vi "Read Pre AIV Values.vi"(8 "error in":errorcluster, 11 "DAC HeatFlow AIV in":refnum<class "DAC HeatFlow AIV.lvclass">) -> (0 "error out":errorcluster, 3 "DAC HeatFlow AIV out":refnum<class "DAC HeatFlow AIV.lvclass">)   [LabVIEW 2019, in "DAC.lvlib" / "DAC HeatFlow AIV.lvclass"]
uses:
  DAC HeatFlow AIV.lvclass
  <vilib>/DAQmx/read.llb/DAQmx Read (Analog DBL 1Chan 1Samp).vi
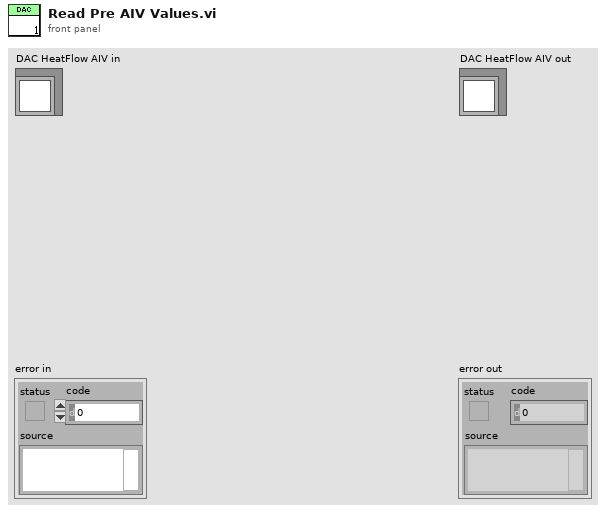
[diagram p1: front panel]
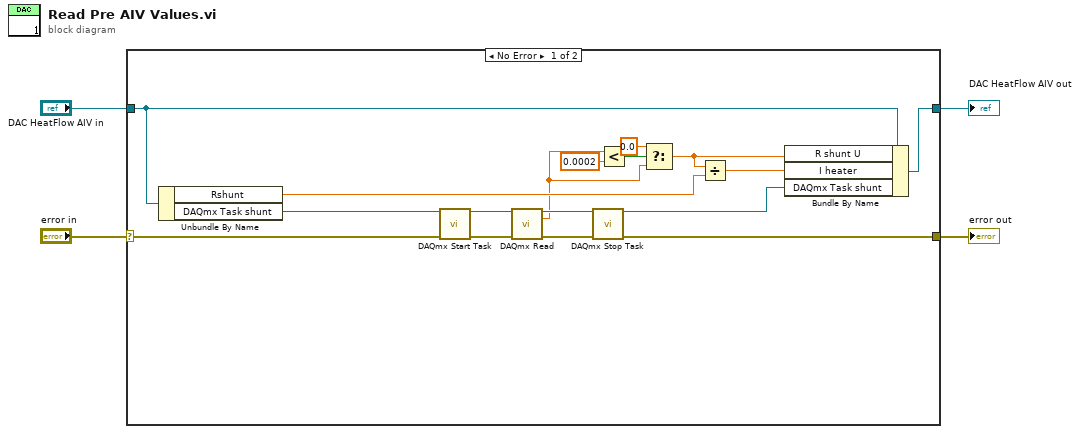
[diagram p0: block diagram]
diagram:
  n1 = case shown="No Error" "error in" {
    selector: "error in" -> [w5 w23]
    tunnel: [w13 w23] -> w3
    tunnel: [w21 w22] -> w1
    tunnel: "DAC HeatFlow AIV in" -> [w20 w22]
    frame No Error {
      n2 = Unbundle By Name(w20) -> ("Rshunt"=w11:dbl, "DAQmx Task shunt"=w19:refnum<k21>)
      n3 = call <vilib>:"DAQmx Start Task.vi"("task/channels in"=w19, "error in"=w5) -> ("task out"=w18:refnum<k21>, "error out"=w15:errorcluster)  [unwired: 12 in]
      n4 = call-poly <vilib>:"DAQmx Read.vi"("task/channels in"=w18, "error in"=w15) -> ("task out"=w17:refnum<k21>, "data"=w7:dbl, "error out"=w14:errorcluster)  [unwired: 11 in]
      n5 = call <vilib>:"DAQmx Stop Task.vi"("task/channels in"=w17, "error in"=w14) -> ("task out"=w16:refnum<k21>, "error out"=w13:errorcluster)  [unwired: 12 in]
      n6 = Less?(x=w7, y=0.0002) -> (x < y?=w9:bool)
      n7 = Select(t=0.0, s=w9, f=w7) -> (s? t:f=w6:dbl)
      n8 = Divide(x=w6, y=w11) -> (x/y=w12:dbl)
      n9 = Bundle By Name(cluster=w20, "R shunt U"=w6, "I heater"=w12, "DAQmx Task shunt"=w16) -> (w21:refnum<class "DAC HeatFlow AIV.lvclass">)
    }
    frame Error {
    }
  }
  "error out" <- w3
  "DAC HeatFlow AIV out" <- w1
